vi "Plenum Fan Control.vi"() -> ()   [LabVIEW 2019]
uses:
  <vilib>/gmath/NI_Gmath.lvlib
panel:
  in  "% Power":dbl min=0.0 max=100.0 step=1.0
  out "Required Voltage":dbl
  in  "stop":bool
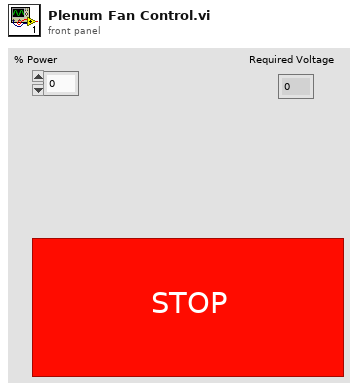
[diagram p1: front panel]
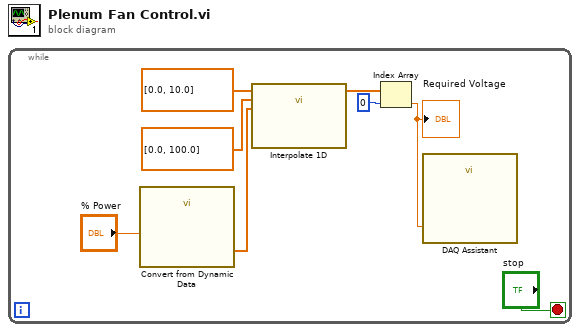
[diagram p0: block diagram]
diagram:
  n1 = while {
    stop <- "stop" stop-if-true
    n2 = call "Convert from Dynamic Data"("Dynamic Data Type"="% Power") -> ("Array"=w7:dbl[])  [unwired: 3 in]
    n3 = call <vilib>:"Interpolate 1D.vi"("xi"=w7, "X"=dbl[] [0.0, 100.0], "Y"=dbl[] [0.0, 10.0]) -> ("yi"=w8:dbl[])  [unwired: 6 in, 2 out]
    n4 = Index Array(array=w8, index=0) -> (element=w2:dbl)
    "Required Voltage" <- w2
    n5 = call "DAQ Assistant"("data"=w2) -> ()  [unwired: 17 in, 2 out]
  }
